vi "Condition Msg VI.vi"(8 "error in":errorcluster, 10 "Ref.Msg VI":refnum<vi>) -> (0 "error out":errorcluster)   [LabVIEW 2025, in "_Msg Rescript.lvlib" / "_Msg Rescript.lvclass"]
uses:
  _Msg Rescript.lvclass
  <vilib>/Utility/traverseref.llb/TRef TravTarget.ctl
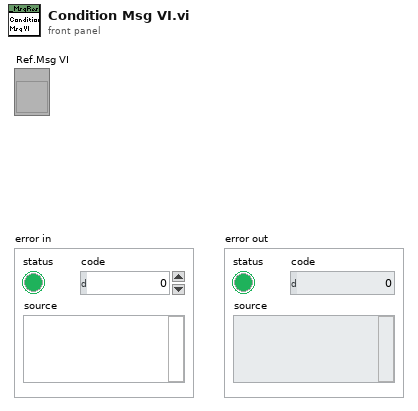
[diagram p1: front panel]
types:
  T1 = typedef "TRef TravTarget.ctl" = enum16{"FP", "BD", "Other"}
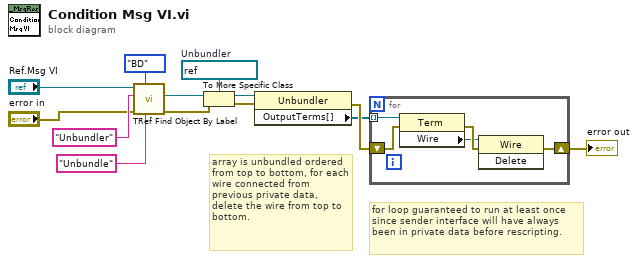
[diagram p0: block diagram]
diagram:
  w11 = refnum<vi> refnum  # Unbundler
  # "for loop guaranteed to run at least once since sender interface will have always been in private data before rescripting."
  # "array is unbundled ordered from top to bottom, for each wire connected from previous private data, delete the wire from top to bottom."
  n1 = call <vilib>:"TRef Find Object By Label.vi"("Label"="Unbundle", "Traverse Target"=TRef_TravTarget."BD", "error in (no error)"="error in", "Class Name"="Unbundler", "VI Ref"="Ref.Msg VI") -> ("error out"=w12:errorcluster, "Found Obj Ref"=w10:refnum<vi>)  [unwired: 3 in, 2 out]
  n2 = To More Specific Class(target class=w11, reference=w10, error in=w12) -> (specific class reference=w7:refnum<vi>, error out=w5:errorcluster)
  n3 = property class="Unbundler"(reference=w7, error in=w5) -> (error out=w13:errorcluster, "OutputTerms[]"=w1:refnum<vi>[])  [unwired: 1 out]
  n4 = for {
    shift-right: [w14] -> w2
    shift-left: w13 -> [w15]
    tunnel: w1 -> [w17] mode=indexing
    n5 = property class="Term"(reference=w17, error in=w15) -> (error out=w18:errorcluster, "Wire"=w16:refnum<vi>)  [unwired: 1 out]
    n6 = invoke class="Wire" method="Delete"(reference=w16, error in=w18) -> (error out=w14:errorcluster)  [unwired: 1 in, 2 out]
  }
  "error out" <- w2
